vi "IMULoop.vi"   [LabVIEW 2015]
uses:
  Common Code/IMU Data.ctl
  navX-MXP Library/COMMON/TypeDefs/Value TypeDefs/navX NAVX_CAL_STATUS.ctl
  navX-MXP Library/COMMON/TypeDefs/Value TypeDefs/navX NAVX_OP_STATUS.ctl
  Robot Global Data.vi
  navX-MXP Library/navX-MXP IMU.lvlib
types:
  T1 = typedef "navX-MXP IMU.lvlib/navX Device TypeDef.ctl" = cluster{"navX Interface Protocol":T2, "navX Interface Protocol TypeDefs":cluster{"SPIDevRef":T3, "I2CDevRef":T5}, "navX System Information":cluster{"Board Information":T7, "Status":T8, "Offsets":T12}, "navX Common Information":cluster{"Update Rate (4Hz-60Hz)":T13, "refnum name":string, "error":errorcluster}}
  T2 = typedef "navX-MXP IMU.lvlib/navX Interface Protocol.ctl" = enum16{"SPI", "I2C"}
  T3 = typedef "WPI_SPIDevRef.ctl" = cluster{"DevStatus":errorcluster, "Handle":i32, "SPI Bus":T4}
  T4 = typedef "spi_bus.ctl" = enum16{"SPI On-Board, CS0", "SPI On-Board, CS1", "SPI On-Board, CS2", "SPI On-Board, CS3", "SPI MXP", "Invalid"}
  T5 = typedef "WPI_I2CDevRef.ctl" = cluster{"DevStatus":errorcluster, "Device Address":u8, "Handle":i32, "I2C Bus":T6}
  T6 = typedef "i2c_bus.ctl" = enum16{"I2C On-Board", "I2C MXP", "Invalid"}
  T7 = typedef "navX-MXP IMU.lvlib/navX Board Information.ctl" = cluster{"WhoAmI (50 | 0x32)":u8, "Board Revision":u8, "Firmware Major Version":u8, "Firmware Minor Version":u8}
  T8 = typedef "navX-MXP IMU.lvlib/navX Status Data.ctl" = cluster{"Update Rate Hz":u8, "Accelerometer Full-Scale Range":u8, "Gyro Full-Scale Range":u16, "NAVX_OP_STATUS":T9, "NAVX_CAL_STATUS":T10, "NAVX_SELFTEST_STATUS":u8, "NAVX_SENSOR_STATUS":T11}
  T9 = typedef "navX-MXP IMU.lvlib/navX NAVX_OP_STATUS.ctl" = u8
  T10 = typedef "navX-MXP IMU.lvlib/navX NAVX_CAL_STATUS.ctl" = u8
  T11 = typedef "navX-MXP IMU.lvlib/navX NAVX_SENSOR_STATUS.ctl" = cluster{"MOVING":bool, "YAW_STABLE":bool, "MAG_DISTURBANCE":bool, "ALTITUDE_VALID":bool, "SEALEVEL_PRESS_SET":bool, "FUSED_HEADING_VALID":bool}
  T12 = typedef "navX-MXP IMU.lvlib/navX Offsets Data.ctl" = cluster{"Yaw":dbl, "Quat W":dbl, "Quat X":dbl, "Quat Y":dbl, "Quat Z":dbl}
  T13 = typedef "navX-MXP IMU.lvlib/navX Update Rate.ctl" = u8
  T14 = typedef "IMU Data.ctl" = cluster{"Pitch":sgl, "Roll":sgl, "Yaw":sgl, "Data Valid?":bool, "Temp":sgl, "MOVING":bool, "YAW_STABLE":bool, "Accel X":sgl, "Accel Y":sgl, "Accel Z":sgl, "Accel Magnitude":sgl, "Pitch Rate":sgl, "Roll Rate":sgl, "Yaw Rate":sgl, "NavX Opened?":bool, "NAVX_CAL_STATUS":T10, "NAVX_OP_STATUS":T9}
  T15 = typedef "navX-MXP IMU.lvlib/navX Vector Data.ctl" = cluster{"X":dbl, "Y":dbl, "Z":dbl}
  T16 = typedef "navX-MXP IMU.lvlib/navX YPRH Data.ctl" = cluster{"Yaw":dbl, "Pitch":dbl, "Roll":dbl, "Heading":dbl}
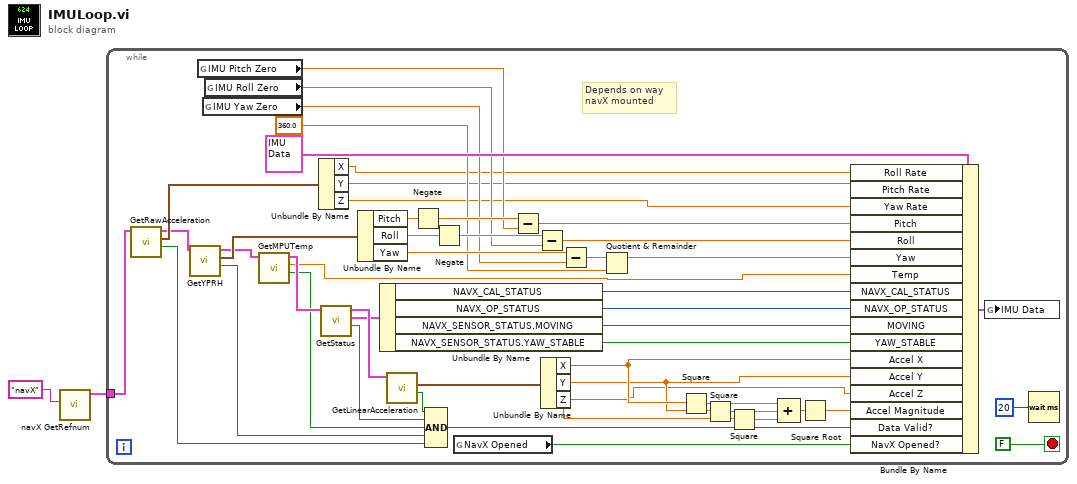
[diagram p0: block diagram]
diagram:
  n1 = call "navX GetRefnum.vi"("refnum name"="navX") -> ("navX Device TypeDef"=w1:T1)  [unwired: 9 in, 1 out]
  n2 = while {
    tunnel: w1 -> [w20]
    stop <- FALSE stop-if-true
    # "Depends on way \nnavX mounted"
    n3 = call "GetRawAcceleration.vi"("navX Device TypeDef"=w20) -> ("Valid?"=w18:bool, "Raw Acceleration"=w19:T15, "navX Device TypeDef"=w17:T1)  [unwired: 8 in]
    n4 = call "GetYPRH.vi"("navX Device TypeDef"=w17) -> ("Valid?"=w15:bool, "YPRH"=w16:T16, "navX Device TypeDef"=w14:T1)  [unwired: 8 in]
    n5 = global read "Robot Global Data.vi" "IMU Pitch Zero"() -> (w44:dbl)
    n6 = global read "Robot Global Data.vi" "IMU Yaw Zero"() -> (w42:dbl)
    n7 = global read "Robot Global Data.vi" "IMU Roll Zero"() -> (w43:dbl)
    n8 = call "GetMPUTemp.vi"("navX Device TypeDef"=w14) -> ("Valid?"=w6:bool, "MPU Temperature (Centigrade)"=w7:dbl, "navX Device TypeDef"=w13:T1)  [unwired: 8 in]
    n9 = Unbundle By Name(w19) -> ("X"=w5:dbl, "Y"=w4:dbl, "Z"=w3:dbl)
    n10 = call "GetStatus.vi"("navX Device TypeDef"=w13) -> ("Valid?"=w11:bool, "Status"=w8:T8, "navX Device TypeDef"=w12:T1)  [unwired: 8 in]
    n11 = Unbundle By Name(w16) -> ("Pitch"=w49:dbl, "Roll"=w48:dbl, "Yaw"=w45:dbl)
    n12 = Unbundle By Name(w8) -> ("NAVX_CAL_STATUS"=w24:T10, "NAVX_OP_STATUS"=w23:T9, "NAVX_SENSOR_STATUS.MOVING"=w22:bool, "NAVX_SENSOR_STATUS.YAW_STABLE"=w21:bool)
    n13 = call "GetLinearAcceleration.vi"("navX Device TypeDef"=w12) -> ("Valid?"=w10:bool, "Linear Acceleration"=w9:T15)  [unwired: 8 in, 1 out]
    n14 = Negate(x=w49) -> (-x=w47:dbl)
    n15 = Compound Arithmetic op=AND(w10, w11, w6, w15, w18) -> (w37:bool)
    n16 = Negate(x=w48) -> (-x=w46:dbl)
    n17 = global read "Robot Global Data.vi" "NavX Opened"() -> (w33:bool)
    n18 = Subtract(x=w47, y=w44) -> (x-y=w41:dbl)
    n19 = Subtract(x=w46, y=w43) -> (x-y=w40:dbl)
    n20 = Unbundle By Name(w9) -> ("X"=w27:dbl, "Y"=w26:dbl, "Z"=w25:dbl)
    n21 = Subtract(x=w45, y=w42) -> (x-y=w39:dbl)
    n22 = Quotient & Remainder(x=w39, y=360.0) -> (x-y*floor(x/y)=w38:dbl)  [unwired: 1 out]
    n23 = Square(x=w27) -> (x^2=w32:dbl)
    n24 = Square(x=w26) -> (x^2=w31:dbl)
    n25 = Square(x=w25) -> (x^2=w30:dbl)
    n26 = Compound Arithmetic op=ADD(w32, w31, w30) -> (w29:dbl)
    n27 = Square Root(x=w29) -> (sqrt(x)=w28:dbl)
    n28 = Bundle By Name(cluster=T14 {"Pitch"=0.0, "Roll"=0.0, "Yaw"=0.0, "Data Valid?"=FALSE, "Temp"=0.0, "MOVING"=FALSE, "YAW_STABLE"=FALSE, "Accel X"=0.0, "Accel Y"=0.0, "Accel Z"=0.0, "Accel Magnitude"=0.0, "Pitch Rate"=0.0, "Roll Rate"=0.0, "Yaw Rate"=0.0, "NavX Opened?"=FALSE, "NAVX_CAL_STATUS"=0, "NAVX_OP_STATUS"=0} ("IMU Data"), "Roll Rate"=w5, "Pitch Rate"=w4, "Yaw Rate"=w3, "Pitch"=w41, "Roll"=w40, "Yaw"=w38, "Temp"=w7, "NAVX_CAL_STATUS"=w24, "NAVX_OP_STATUS"=w23, "MOVING"=w22, "YAW_STABLE"=w21, "Accel X"=w27, "Accel Y"=w26, "Accel Z"=w25, "Accel Magnitude"=w28, "Data Valid?"=w37, "NavX Opened?"=w33) -> (w50:T14)
    n29 = global write "Robot Global Data.vi" "IMU Data"(w50) -> ()
    n30 = Wait (ms)(milliseconds to wait=u32 20) -> ()  [unwired: 1 out]
  }
